vi "testTCPIPgraph.vi"() -> ()   [LabVIEW 2013]
panel:
  out "Waveform Graph 2":dbl[](graph)
  out "Waveform Graph":dbl[](graph)
  out "error out":errorcluster
  in  "stop 2":bool
  in  "Mode":T1(ring)=enum."CRLF"
  out "Caractères reçus":string
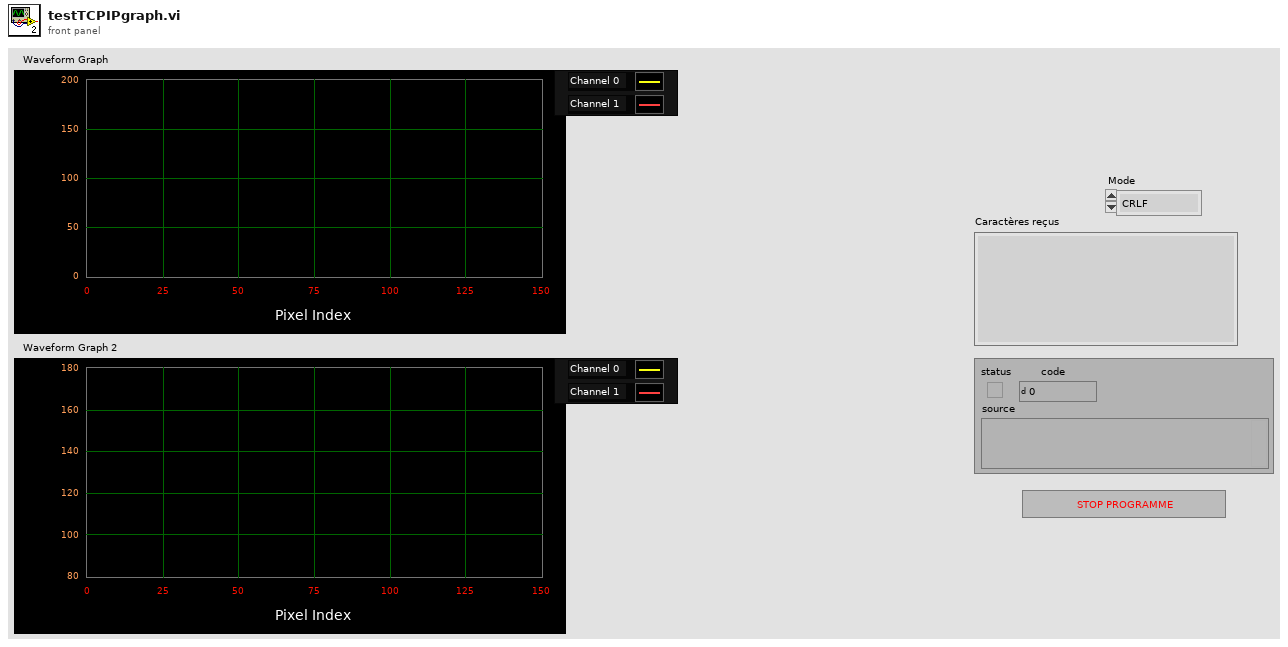
[diagram p1: front panel]
types:
  T1 = enum16{"Standard", "Buffered", "CRLF", "Immediate"}
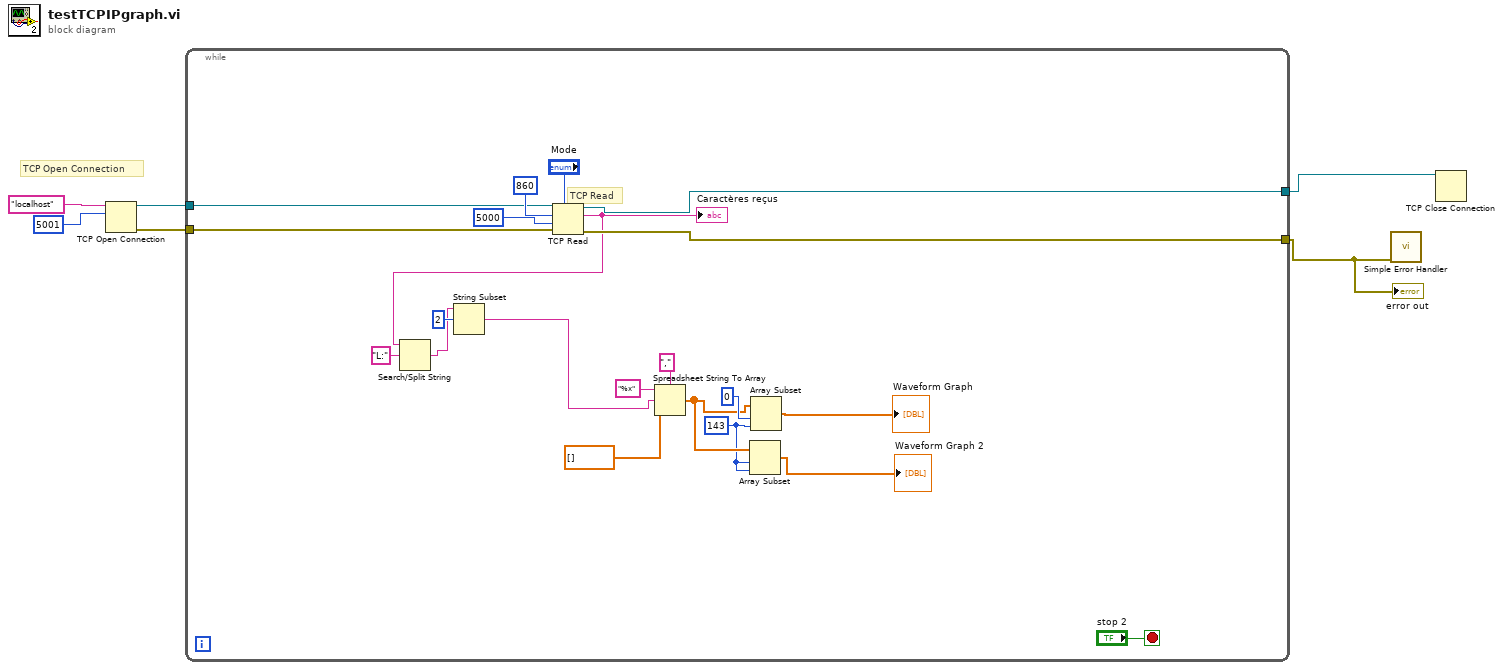
[diagram p0: block diagram]
diagram:
  # "TCP Open Connection"
  n1 = TCP Open Connection(address="localhost", remote port or service name=u16 5001) -> (connection ID=w4:refnum<k5>, error out=w3:errorcluster)  [unwired: 3 in]
  n2 = while {
    tunnel: w4 -> [w23]
    tunnel: w3 -> [w22]
    tunnel: [w21] -> w1
    tunnel: [w20] -> w2
    stop <- "stop 2" stop-if-true
    w7 = 143 ("length")
    # "TCP Read"
    n3 = TCP Read(connection ID=w23, bytes to read=860, error in (no error)=w22, 7:"Mode", 9:5000 ("timeout ms (25000)")) -> (connection ID out=w20:refnum<k5>, data out=w15:string, error out=w21:errorcluster)
    "Caractères reçus" <- w15
    n4 = Search/Split String(string=w15, search string/char (-)="L:") -> (match + rest of string=w17:string)  [unwired: 1 in, 2 out]
    n5 = String Subset(string=w17, offset (0)=2) -> (substring=w16:string)  [unwired: 1 in]
    n6 = Spreadsheet String To Array(delimiter (Tab)=",", format string="%x", spreadsheet string=w16, array type (2D Dbl)=dbl[] []) -> (array=w8:dbl[])
    n7 = Array Subset(array=w8, index=w7, length=w7) -> (→"Waveform Graph 2":dbl[])
    n8 = Array Subset(array=w8, index=0, length=w7) -> (→"Waveform Graph":dbl[])
  }
  "error out" <- w1
  n9 = call <vilib>:"Simple Error Handler.vi"("error in (no error)"=w1) -> ()  [unwired: 4 in, 5 out]
  n10 = TCP Close Connection(connection ID=w2) -> ()  [unwired: 2 in, 2 out]
